vi "Write Display Function.vi"(8 "error in (no error)":errorcluster, 9 "Display Function":T1, 10 "VISA resource name in":refnum<visa-resource-name>, 11 "LCD-I2C in":refnum<class "LCD-I2C.lvclass">) -> (0 "error out":errorcluster, 2 "VISA resource name":refnum<visa-resource-name>, 3 "LCD-I2C out":refnum<class "LCD-I2C.lvclass">)   [LabVIEW 2023, in "CTI-Visa-DeviceLib.lvlib" / "LCD-I2C.lvclass"]
uses:
  LCD-I2C.lvclass
  Display Function.ctl
  Bus Mode.ctl
  Lines.ctl
  Glyph Size.ctl
  Command.ctl
  LCD-I2C.lvclass/LCD-I2C.ctl
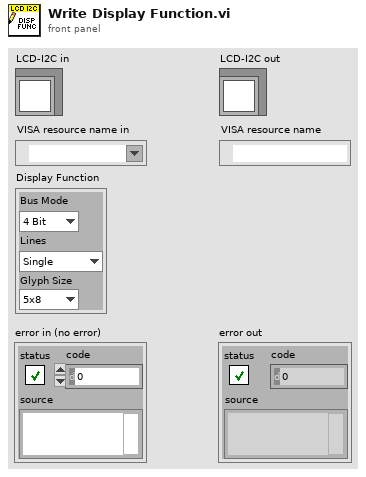
[diagram p1: front panel]
types:
  T1 = typedef "CTI-Visa-DeviceLib.lvlib/LCD-I2C.lvclass/Display Function.ctl" = cluster{"Bus Mode":T2, "Lines":T3, "Glyph Size":T4}
  T2 = typedef "CTI-Visa-DeviceLib.lvlib/LCD-I2C.lvclass/Bus Mode.ctl" = enum8{"4 Bit", "8 Bit"}
  T3 = typedef "CTI-Visa-DeviceLib.lvlib/LCD-I2C.lvclass/Lines.ctl" = enum8{"Single", "Multiline"}
  T4 = typedef "CTI-Visa-DeviceLib.lvlib/LCD-I2C.lvclass/Glyph Size.ctl" = enum8{"5x8", "5x10"}
  T5 = typedef "CTI-Visa-DeviceLib.lvlib/LCD-I2C.lvclass/Command.ctl" = enum16{"Clear Display", "Return Home", "Entry Mode Set", "Display Control", "Cursor Shift", "Function Set", "Set CGRAM Addr", "Set DDRAM Addr"}
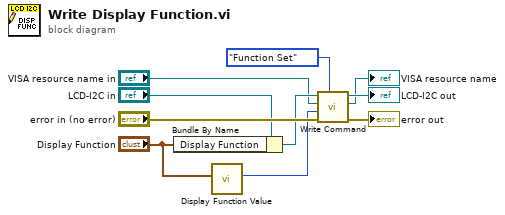
[diagram p0: block diagram]
diagram:
  n1 = Bundle By Name(cluster="LCD-I2C in", "Display Function"="Display Function") -> (w7:refnum<class "LCD-I2C.lvclass">)
  n2 = call "Display Function Value.vi"("Display Function"="Display Function") -> ("DisplayFunc"=w3:u8)  [unwired: 10 in]
  n3 = call "Write Command.vi"("Command"=Command."Function Set", "error in (no error)"="error in (no error)", "Value"=w3, "VISA resource name in"="VISA resource name in", "LCD-I2C in"=w7) -> ("error out"=→"error out":errorcluster, "VISA resource name"=→"VISA resource name":refnum<visa-resource-name>, "LCD-I2C out"=→"LCD-I2C out":refnum<class "LCD-I2C.lvclass">)  [unwired: 4 in]
